vi "NStageMRate Decimation (FPGA).vi"() -> ()   [LabVIEW 2012]
uses:
  <vilib>/rvi/Emulation/niFpgaSctlEmulationGetInTimedLoop.vi
  <vilib>/rvi/DataTransferAndStorage/Container/Common/niFpgaContainerGetUniqueNameForEmu.vi
  <vilib>/rvi/FIFO/Fifo_Resource/nirvififoEmulationSetSize.vi
  <vilib>/rvi/Emulation/niFpgaSctlEmulationFifoFullMgr.vi
  <vilib>/rvi/errors/niFpgaSetErrorForExecOnDevCompSimple.vi
  <vilib>/rvi/eio/common/nirviEmuReportErrorAndStop.vi
  <vilib>/rvi/interface/RandomDataEmulation/nirviRandomDataFPGAFIFO.vi
  <vilib>/rvi/interface/RandomDataEmulation/niFpgaRandomDataHandleErrors.vi
  Instance           1 36Saved   NStageMRateDecimation (FPGA) .vi
  <vilib>/rvi/eio/common/nirviEmuTemplateMethod_errors.vi
  <vilib>/rvi/Emulation/niFpgaSctlEmulationResourceMgr.vi
  <vilib>/rvi/DataTransferAndStorage/Container/XNode/niFpgaContainer.xnode
  <vilib>/rvi/FIFO/Fifo_Resource/nirvififoEmulationRead.vi
  <vilib>/rvi/interface/RandomDataEmulation/nirviRandomDataFpgaReadWriteTemplate.vi
  <vilib>/eio/EIONode/EIONode.xnode
  <vilib>/rvi/FIFO/Fifo_Resource/nirvififoEmulationWrite.vi
panel:
  out "Filtered Signals":T1(graph)
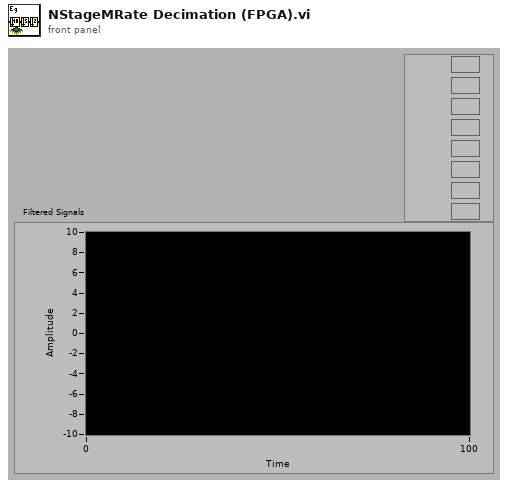
[diagram p1: front panel]
types:
  T1 = cluster{"[0]":u32, "[1]":u32, "[2]":u32, "[3]":u32, "[4]":u32, "[5]":u32, "[6]":u32, "[7]":u32, "[8]":u32}
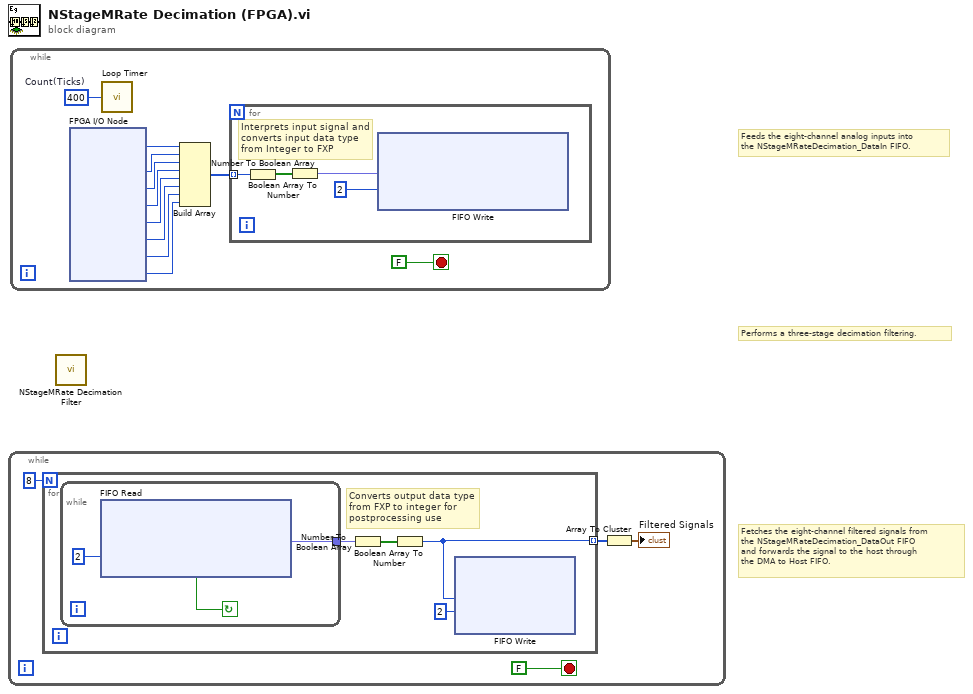
[diagram p0: block diagram]
diagram:
  # "Fetches the eight-channel filtered signals from\nthe NStageMRateDecimation_DataOut FIFO\nand forwards the signal to the host through\nthe DMA to Host FIFO."
  # "Performs a three-stage decimation filtering."
  # "Feeds the eight-channel analog inputs into\nthe NStageMRateDecimation_DataIn FIFO."
  n1 = while {
    stop <- FALSE stop-if-true
    n2 = for {
      N: 8 -> [_]
      tunnel: [w5] -> w3 mode=indexing
      # "Converts output data type\nfrom FXP to integer for\npostprocessing use"
      n3 = while {
        tunnel: [w9] -> w6
        stop <- w10 continue-if-true
        n4 = xnode ("FIFO Read")("Timeout"=2) -> ("Element"=w9:fxp<+/-,16,4>, "Timed Out?"=w10:bool)  [unwired: 1 in, 1 out]
      }
      n5 = Number To Boolean Array(number=w6) -> (Boolean array=w7:bool[])
      n6 = Boolean Array To Number(Boolean array=w7) -> (number=w5:u32)
      n7 = xnode ("FIFO Write")("Element"=w5, "Timeout"=2) -> ()  [unwired: 1 in, 2 out]
    }
    n8 = Array To Cluster(array=w3) -> (cluster=→"Filtered Signals":T1)
  }
  n9 = while {
    stop <- FALSE stop-if-true
    w22 = u16 400  # Count(Ticks)
    n10 = xnode "FPGA I/O Node"() -> ("AI0"=w21:i16, "AI1"=w18:i16, "AI2"=w17:i16, "AI3"=w16:i16, "AI4"=w15:i16, "AI5"=w14:i16, "AI6"=w13:i16, "AI7"=w12:i16)  [unwired: 8 in, 8 out]
    n11 = call "Loop Timer"("Count(Ticks)"=w22) -> ()  [unwired: 1 out]
    n12 = Build Array(w21, w18, w17, w16, w15, w14, w13, w12) -> (w20:i16[])
    n13 = for {
      tunnel: w20 -> [w24] mode=indexing
      # "Interprets input signal and \nconverts input data type \nfrom Integer to FXP"
      n14 = Number To Boolean Array(number=w24) -> (Boolean array=w25:bool[])
      n15 = Boolean Array To Number(Boolean array=w25) -> (number=w23:fxp<+/-,16,1>)
      n16 = xnode ("FIFO Write")("Element"=w23, "Timeout"=2) -> ()  [unwired: 1 in, 2 out]
    }
  }
  n17 = call "NStageMRate Decimation Filter.vi"() -> ()  [unwired: 1 out]
